vi "SimpleStreamFullSpectrumToStorageExample.vi"() -> ()   [LabVIEW 2016]
uses:
  h.Library/COMM/CTL/h.COMM.Socket Type.ctl
  h.Library.lvlib
panel:
  out "Status String":string
  out "error out":errorcluster
  in  "IP Address":string="10.0.41.3"
  out "Status":i32(slide) scale=0.0..100.0
  in  "Number of Seconds to Acquire":i32=5
  in  "Data Rate Divider":i32=1
  in  "Number of Averages":i32=1
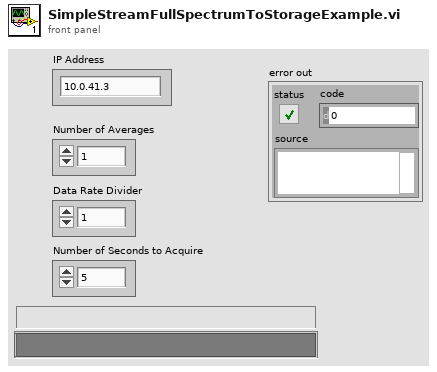
[diagram p1: front panel]
types:
  T1 = typedef "h.Library.lvlib/h.COMM.Socket Type.ctl" = u16
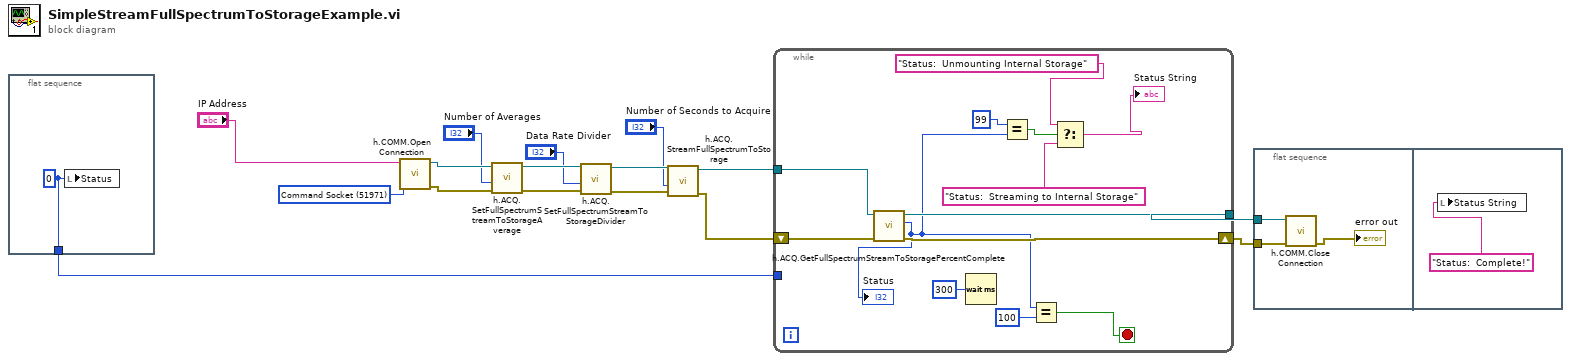
[diagram p0: block diagram]
diagram:
  w15 = T1 51971 items=["Command Socket"=51971, "Streaming Peak Data Socket"=51972, "Streaming Spectral Data Socket"=51973] ("Port")
  n1 = flat-sequence {
    tunnel: [w17] -> w1
    frame #0 {
      w17 = 0 ("Status")
      n2 = local write "Status"(w17) -> ()
    }
  }
  n3 = call "h.COMM.Open Connection.vi"("Port"=w15, "Address"="IP Address") -> ("error out"=w12:errorcluster, "Connection ID"=w14:refnum<k5>)  [unwired: 8 in]
  n4 = call "h.ACQ.SetFullSpectrumStreamToStorageAverage.vi"("error in"=w12, "Number of Averages"="Number of Averages", "Connection ID In"=w14) -> ("error out"=w11:errorcluster, "Connection ID Out"=w10:refnum<k5>)  [unwired: 7 in]
  n5 = call "h.ACQ.SetFullSpectrumStreamToStorageDivider.vi"("error in"=w11, "Data Rate Divider"="Data Rate Divider", "Connection ID In"=w10) -> ("error out"=w6:errorcluster, "Connection ID Out"=w8:refnum<k5>)  [unwired: 7 in]
  n6 = call "h.ACQ.StreamFullSpectrumToStorage.vi"("error in"=w6, "Seconds to Acquire"="Number of Seconds to Acquire", "Connection ID In"=w8) -> ("error out"=w5:errorcluster, "Connection ID Out"=w4:refnum<k5>)  [unwired: 7 in]
  n7 = while {
    shift-right: [w24] -> w2
    shift-left: w5 -> [w30]
    tunnel: w4 -> [w29]
    tunnel: [w25] -> w3
    tunnel: w1 -> [_]
    stop <- w26 stop-if-true
    n8 = call "h.ACQ.GetFullSpectrumStreamToStoragePercentComplete.vi"("error in"=w30, "Connection ID"=w29) -> ("error out"=w24:errorcluster, "Percent Complete"=w22:i32, "Connection ID out"=w25:refnum<k5>)  [unwired: 7 in]
    "Status" <- w22
    n9 = Wait (ms)(milliseconds to wait=u32 300) -> ()  [unwired: 1 out]
    n10 = Equal?(x=99 ("y"), y=w22) -> (x = y?=w21:bool)
    n11 = Equal?(x=w22, y=100) -> (x = y?=w26:bool)
    n12 = Select(t="Status:  Unmounting Internal Storage", s=w21, f="Status:  Streaming to Internal Storage") -> (s? t:f=→"Status String":string)
  }
  n13 = flat-sequence {
    tunnel: w3 -> [w33]
    tunnel: w2 -> [w31]
    frame #0 {
      n14 = call "h.COMM.Close Connection.vi"("error in"=w31, "Connection ID"=w33) -> ("error out"=→"error out":errorcluster)  [unwired: 9 in]
    }
    frame #1 {
      n15 = local write "Status String"("Status:  Complete!") -> ()
    }
  }
